vi "Sandfall.vi"() -> ()   [LabVIEW 2018]
uses:
  <vilib>/picture/picture.llb/Draw True-Color Pixmap.vi
panel:
  out "new picture":picture
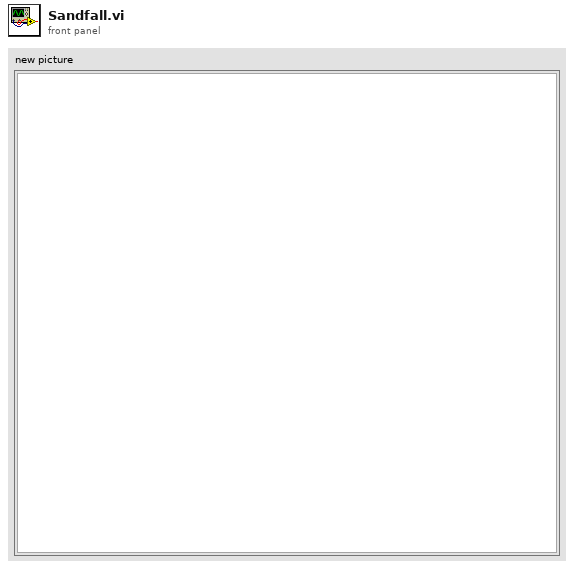
[diagram p1: front panel]
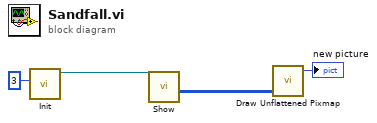
[diagram p0: block diagram]
diagram:
  n1 = call "Init.vi"("Depth"=3) -> ("Picture out"=w3:refnum<class "Picture.lvclass">)  [unwired: 10 in]
  n2 = call "Show.vi"("Picture in"=w3) -> ("Pixmap 2D"=w2:u32[][])  [unwired: 9 in, 1 out]
  n3 = call-poly <vilib>:"Draw Unflattened Pixmap.vi"("data (RGB format)"=w2) -> ("new picture"=→"new picture":picture)  [unwired: 8 in]
